vi "LINX - Digital Write Benchmark.vi"() -> ()   [LabVIEW 2019]
uses:
  <vilib>/MakerHub/LINX/Public/Peripherals/Digital/Digital Write 1 Chan.vi
  <vilib>/MakerHub/LINX/Public/Peripherals/Digital/Digital Write N Chans.vi
  <vilib>/MakerHub/LINX/Private/Local IO/LinxDigitalWrite.vi
  <vilib>/MakerHub/LINX/Public/Utilities/Check Channel.vi
  <vilib>/MakerHub/LINX/Public/Utilities/Open Local.vi
  <vilib>/MakerHub/LINX/Private/Utilties/Generate Error.vi
  <vilib>/MakerHub/LINX/LMH-LINX.lvlib
panel:
  in  "Warmup Iterations":i32=100
  out "Chart":dbl(graph)
  in  "Stop Button":bool
  in  "Benchmark Iterations":i32=1000
  out "Samples Per Second":i32
  in  "DO Channel":u8=7
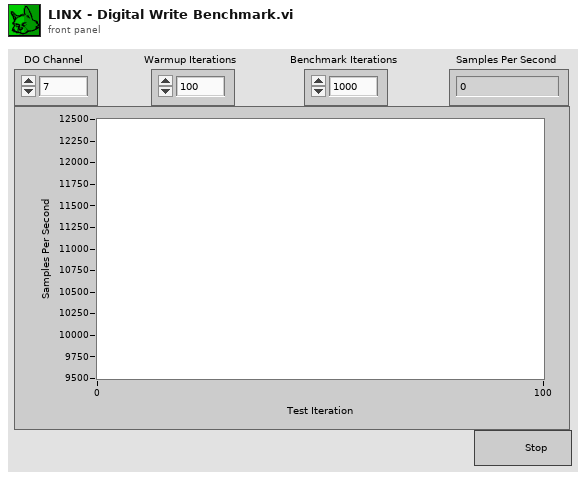
[diagram p1: front panel]
types:
  T1 = typedef "LMH-LINX.lvlib/LINX Ref.ctl" = cluster{"IO":T2, "Interface":T3, "LINX Device Config":T4}
  T2 = typedef "LMH-LINX.lvlib/Platform.ctl" = enum16{"Remote", "Local"}
  T3 = typedef "LMH-LINX.lvlib/Interface.ctl" = enum16{"Serial", "TCP"}
  T4 = typedef "LMH-LINX.lvlib/Device.lvlib/LINX Device Config.ctl" = cluster{"Interface":T3, "COM Port":refnum<visa-resource-name>, "TCP Configuration":T5, "Device Family":u8, "Device ID":u8, "Device Name":string, "TCP Ref":refnum<k5>, "Channels":T6}
  T5 = typedef "LMH-LINX.lvlib/Device.lvlib/TCP Config.ctl" = cluster{"IP Address":string, "Port":u16}
  T6 = typedef "LMH-LINX.lvlib/Channels.ctl" = cluster{"DI":u8[], "DO":u8[], "AI":u8[], "AO":u8[], "PWM":u8[], "QE":u8[], "UART":u8[], "I2C 2":u8[], "SPI":u8[], "CAN":u8[], "Servo":u8[], "AI Ref (V)":dbl, "AI Resolution (Bits)":u8, "AO Ref (V)":dbl, "AO Resolution (Bits)":u8}
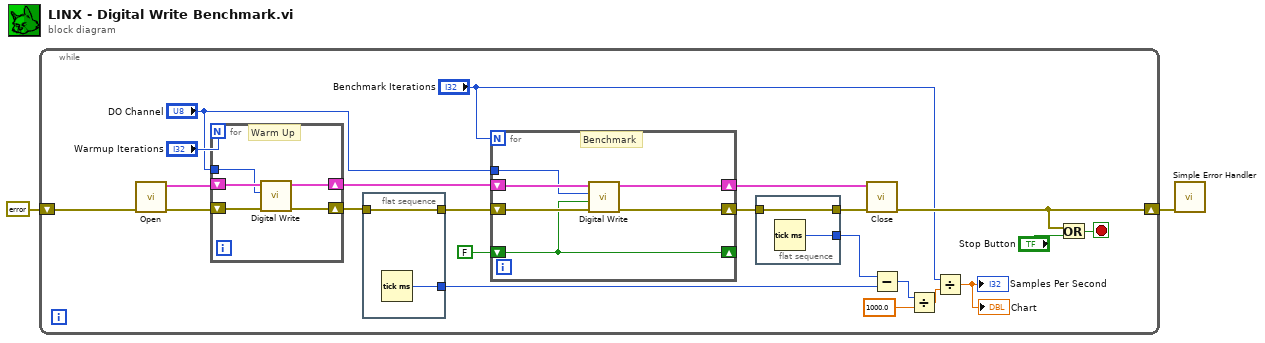
[diagram p0: block diagram]
diagram:
  n1 = while {
    shift-right: [w14] -> w2
    shift-left: errorcluster {"status"=FALSE, "code"=0, "source"=""} ("Error Out") -> [w12]
    stop <- w3 stop-if-true
    n2 = call-poly <vilib>:"Open.vi"("Error In"=w12) -> ("Error Out"=w19:errorcluster, "LINX Resource"=w20:T1)  [unwired: 8 in, 1 out]
    n3 = for {
      N: "Warmup Iterations" -> [_]
      shift-right: [w27] -> w17
      shift-left: w20 -> [w29]
      shift-right: [w26] -> w18
      shift-left: w19 -> [w28]
      tunnel: "DO Channel" -> [w25]
      # "Warm Up"
      n4 = call-poly <vilib>:"Digital Write.vi"("Error In"=w28, "DO Channel"=w25, "LINX Resource"=w29) -> ("Error Out"=w26:errorcluster, "LINX Resource"=w27:T1)  [unwired: 7 in]
    }
    n5 = flat-sequence {
      tunnel: [w39] -> w23
      tunnel: w18 -> [w39]
      tunnel: [w38] -> w6
      frame #0 {
        n6 = Tick Count (ms)() -> (millisecond timer value=w38:u32)
      }
    }
    n7 = for {
      N: "Benchmark Iterations" -> [_]
      shift-right: [w33] -> w24
      shift-left: w17 -> [w35]
      shift-right: [w32] -> w22
      shift-left: w23 -> [w34]
      tunnel: "DO Channel" -> [w31]
      shift-right: [w30] -> _
      shift-left: FALSE ("x") -> [w30]
      # "Benchmark"
      n8 = call-poly <vilib>:"Digital Write.vi"("Error In"=w34, "Output Value"=w30, "DO Channel"=w31, "LINX Resource"=w35) -> ("Error Out"=w32:errorcluster, "LINX Resource"=w33:T1)  [unwired: 6 in]
    }
    n9 = flat-sequence {
      tunnel: [w37] -> w21
      tunnel: w22 -> [w37]
      tunnel: [w36] -> w7
      frame #0 {
        n10 = Tick Count (ms)() -> (millisecond timer value=w36:u32)
      }
    }
    n11 = call <vilib>:"Close.vi"("Error In"=w21, "LINX Resource"=w24) -> ("Error Out"=w14:errorcluster)  [unwired: 9 in]
    n12 = Subtract(x=w7, y=w6) -> (x-y=w10:u32)
    n13 = Divide(x=w10, y=1000.0) -> (x/y=w9:dbl)
    n14 = Divide(x="Benchmark Iterations", y=w9) -> (x/y=→"Chart" →"Samples Per Second":dbl)
    n15 = Or(x=w14, y="Stop Button") -> (x .or. y?=w3:bool)
  }
  n16 = call <vilib>:"Simple Error Handler.vi"("error in (no error)"=w2) -> ()  [unwired: 4 in, 5 out]
